vi "Add Buffers with Children.vi"(4 "channels":T1[](array[typedef]) {"string offset" format="%d bytes"}, 5 "inline":bool, 6 "Decimation":u64, 7 "Transfer Group Status":refnum<class "Status.lvclass">, 8 "error in (no error)":errorcluster, 9 "Buffers":refnum<class "Buffers.lvclass">, 10 "parent tag":string, 11 "Application Data In":T4) -> (0 "error out":errorcluster, 3 "Application Data out":T4)   [LabVIEW 2017, in "DSF Core.lvlib"]
uses:
  DSF Core.lvlib
  Main VI/Application Data.ctl
  <vilib>/NI/Memory Manager/Classes/Pointer/Pointer.lvclass
  Classes/Framework/Framework.lvclass
  Buffer Reader/Buffer Data.ctl
  Classes/Buffer/Buffer.lvclass
  C:/Program Files (x86)/National Instruments/LabVIEW 2017/vi.lib/NI/Memory Manager/Classes/Pointer/Pointer.lvclass
  Classes/Transfer Group Status/Status.lvclass
  Typedefs/DSF Engine Framework Configuration.ctl
  Typedefs/DSF Engine Plugin Configuration.ctl
  Typedefs/DSF Timing Info.ctl
  Typedefs/DSF Engine Plugin Thread Configuration.ctl
  Typedefs/DSF Settings Info.ctl
  Typedefs/DSF Engine Transfer Group Configuration.ctl
  Typedefs/DSF Direction.ctl
  Typedefs/DSF Engine Transfer Configuration.ctl
  Typedefs/DSF Byte Order.ctl
  Typedefs/DSF Engine Channel Configuration.ctl
  Typedefs/DSF Data Type.ctl
  Typedefs/DSF Timeout Behavior.ctl
  Classes/Buffers/Buffers.lvclass
  ID to Tree Items/Tree Item Type.ctl
  Classes/Buffers/Buffers.lvclass/Buffers.ctl
  <vilib>/NI/Memory Manager/Classes/Pointer/Pointer.lvclass/Pointer.ctl
  Classes/Buffer/Get Buffer Size.vi
  Sizeof.vi
  <vilib>/NI/Memory Manager/Classes/Pointer/Get Size.vi
  Classes/Buffer/Subset Buffer.vi
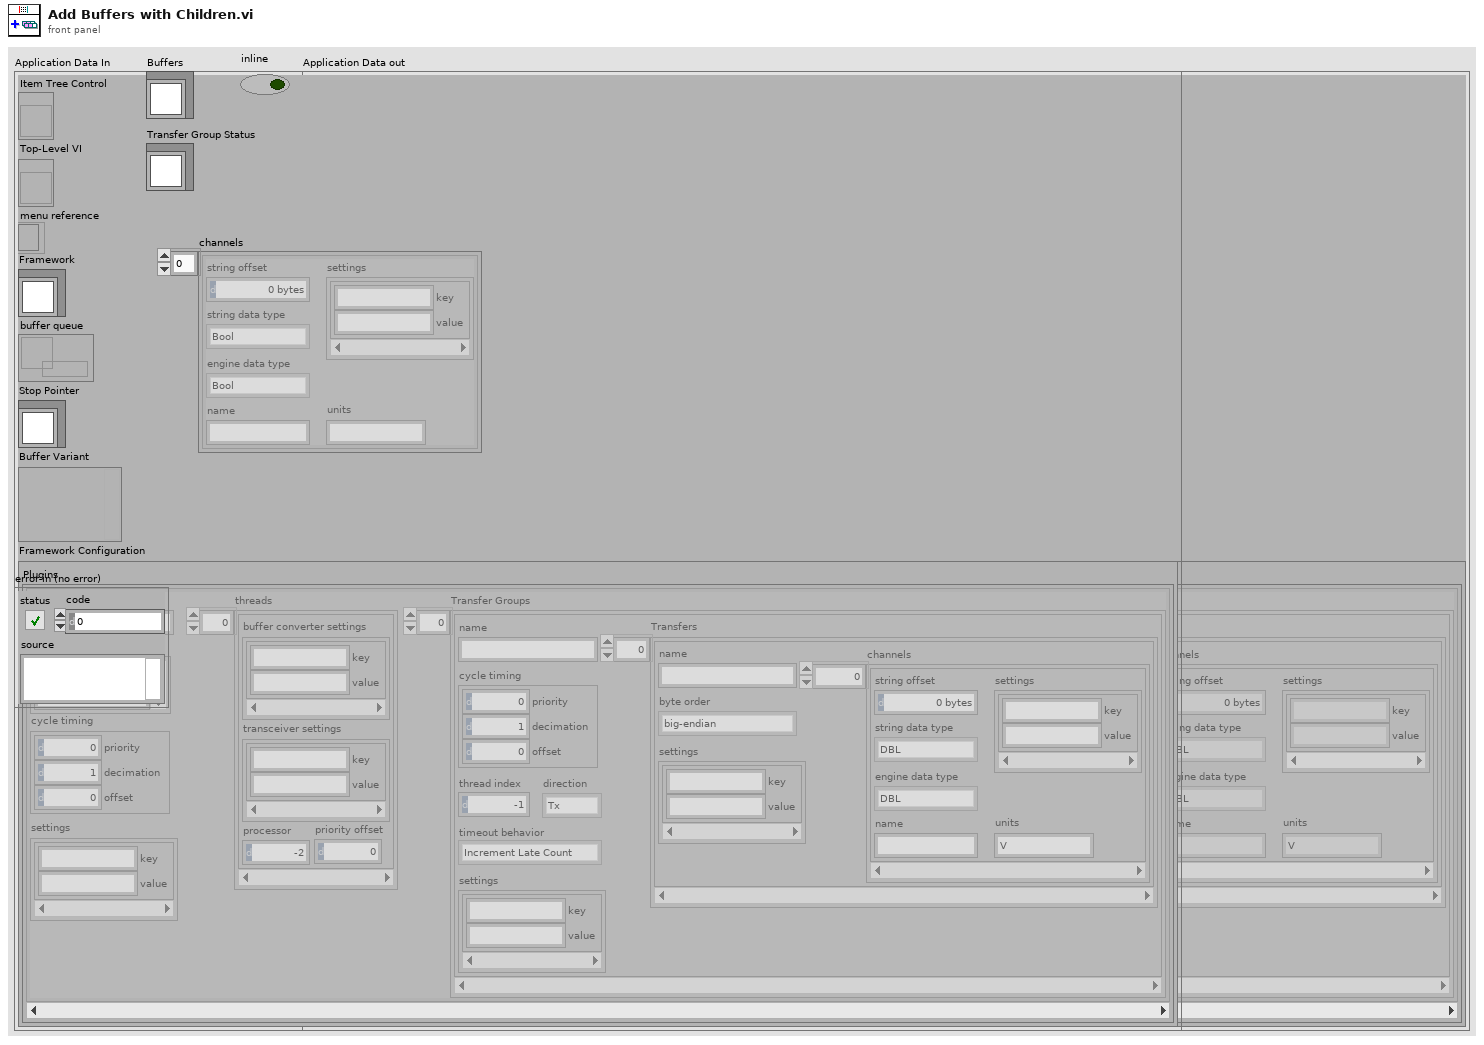
[diagram p1: front panel]
types:
  T1 = typedef "DSF Core.lvlib/DSF Engine Channel Configuration.ctl" = cluster{"string offset":u64, "string data type":T2, "engine data type":T2, "name":string, "settings":T3, "units":string}
  T2 = typedef "DSF Core.lvlib/DSF Data Type.ctl" = enum8{"Bool", "SGL", "DBL", "I8", "I16", "I32", "I64", "U8", "U16", "U32", "U64"}
  T3 = typedef "DSF Core.lvlib/DSF Settings Info.ctl" = cluster{"key":string, "value":string}[]
  T4 = typedef "DSF Core.lvlib/Application Data.ctl" = cluster{"Item Tree Control":refnum<vi>, "Top-Level VI":refnum<vi>, "menu reference":refnum<k9>, "Framework":refnum<class "Framework.lvclass">, "buffer queue":refnum<queue>, "Stop Pointer":refnum<class "Pointer.lvclass">, "Buffer Variant":variant, "Framework Configuration":T5}
  T5 = typedef "DSF Core.lvlib/DSF Engine Framework Configuration.ctl" = cluster{"Plugins":T6[]}
  T6 = typedef "DSF Core.lvlib/DSF Engine Plugin Configuration.ctl" = cluster{"name":string, "components":string[], "cycle timing":T7, "threads":T8[], "Transfer Groups":T9[], "settings":T3}
  T7 = typedef "DSF Core.lvlib/DSF Timing Info.ctl" = cluster{"priority":u64, "decimation":u64, "offset":u64}
  T8 = typedef "DSF Core.lvlib/DSF Engine Plugin Thread Configuration.ctl" = cluster{"buffer converter settings":T3, "transceiver settings":T3, "processor":i32, "priority offset":i16}
  T9 = typedef "DSF Core.lvlib/DSF Engine Transfer Group Configuration.ctl" = cluster{"name":string, "direction":T10, "cycle timing":T7, "thread index":i32, "settings":T3, "Transfers":T11[], "timeout behavior":T13}
  T10 = typedef "DSF Core.lvlib/DSF Direction.ctl" = enum8{"Tx", "Rx"}
  T11 = typedef "DSF Core.lvlib/DSF Engine Transfer Configuration.ctl" = cluster{"name":string, "byte order":T12, "settings":T3, "channels":T1[]}
  T12 = typedef "DSF Core.lvlib/DSF Byte Order.ctl" = enum8{"big-endian", "little-endian"}
  T13 = typedef "DSF Core.lvlib/DSF Timeout Behavior.ctl" = enum8{"Increment Late Count", "Throw Error"}
  T14 = typedef "DSF Core.lvlib/Buffer Data.ctl" = cluster{"Buffer":refnum<class "Buffer.lvclass">, "Status":refnum<class "Status.lvclass">, "decimation":u64, "avg bandwidth":dbl}
  T15 = typedef "DSF Core.lvlib/Tree Item Type.ctl" = enum16{"Framework", "Plugin Group", "Plugin", "Group", "Transfer", "Buffer", "Channel"}
  T16 = typedef "DSF Core.lvlib/Tree Item.ctl" = cluster{"Left Cell String":string, "Child Text":string[], "Child Tag":string, "Glyph Index":i32}
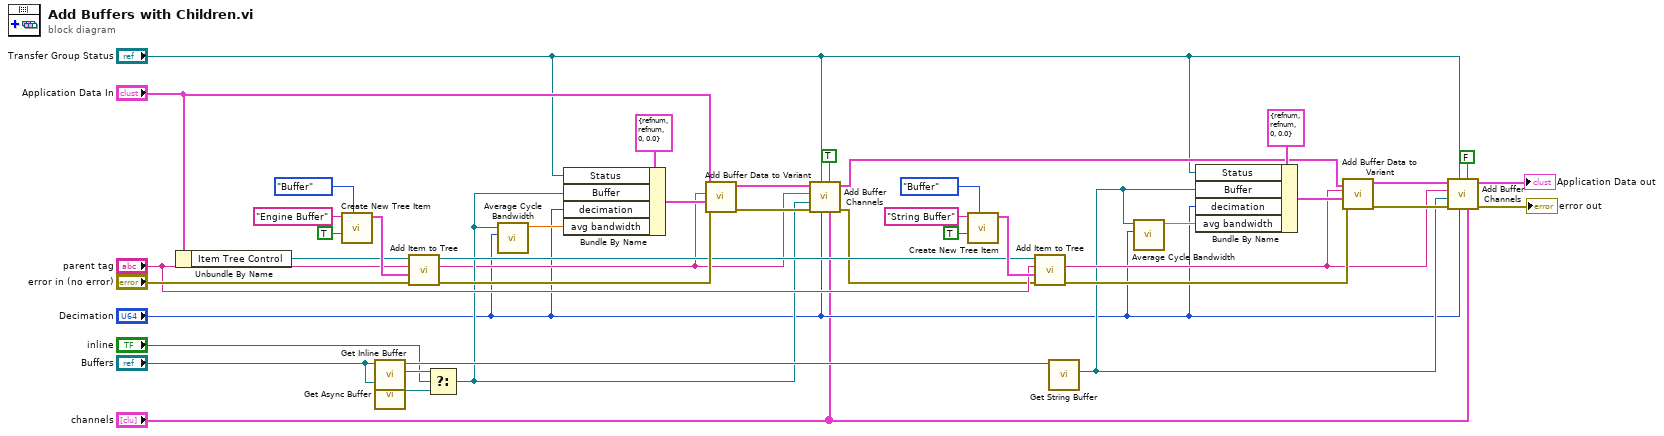
[diagram p0: block diagram]
diagram:
  n1 = Unbundle By Name("Application Data In") -> ("Item Tree Control"=w25:refnum<vi>)
  n2 = call "Create New Tree Item.vi"("Item Type"=Tree_Item_Type."Buffer", "found?"=TRUE, "Left Cell String"="Engine Buffer") -> ("Item"=w27:T16)  [unwired: 7 in, 1 out]
  n3 = call "Get Inline Buffer.vi"("Buffers in"="Buffers") -> ("Inline Buffer"=w19:refnum<class "Buffer.lvclass">, "Buffers out"=w34:refnum<class "Buffers.lvclass">)  [unwired: 9 in]
  n4 = call "Get Async Buffer.vi"("Buffers in"="Buffers") -> ("Async Buffer"=w20:refnum<class "Buffer.lvclass">)  [unwired: 9 in, 1 out]
  n5 = call "Add Item to Tree.vi"("error in (no error)"="error in (no error)", "Item"=w27, "parent tag"="parent tag", "TreeControl in"=w25) -> ("error out"=w40:errorcluster, "new item tag"=w12:string, "TreeControl out"=w35:refnum<vi>)  [unwired: 5 in]
  n6 = Select(t=w19, s="inline", f=w20) -> (s? t:f=w13:refnum<class "Buffer.lvclass">)
  n7 = call "Average Cycle Bandwidth.vi"("Decimation"="Decimation", "Buffer"=w13) -> ("avergage cycle bandwidth"=w23:dbl)  [unwired: 9 in]
  n8 = Bundle By Name(cluster=T14 {"Buffer"=refnum, "Status"=refnum, "decimation"=0, "avg bandwidth"=0.0} ("Buffer data"), "Status"="Transfer Group Status", "Buffer"=w13, "decimation"="Decimation", "avg bandwidth"=w23) -> (w39:T14)
  n9 = call "Add Buffer Data to Variant.vi"("error in (no error)"=w40, "Buffer data"=w39, "tag"=w12, "Application Data In in"="Application Data In") -> ("error out"=w15:errorcluster, "Application Data In out"=w17:T4)  [unwired: 6 in]
  n10 = call "Add Buffer Channels.vi"("channels"="channels", "engine (T) / string (F)"=TRUE, "Decimation"="Decimation", "Transfer Group Status"="Transfer Group Status", "error in (no error)"=w15, "Buffer"=w13, "parent tag"=w12, "Application Data In"=w17) -> ("error out"=w14:errorcluster, "Application Data out"=w16:T4)  [unwired: 2 in]
  n11 = call "Create New Tree Item.vi"("Item Type"=Tree_Item_Type."Buffer", "found?"=TRUE, "Left Cell String"="String Buffer") -> ("Item"=w36:T16)  [unwired: 7 in, 1 out]
  n12 = call "Add Item to Tree.vi"("error in (no error)"=w14, "Item"=w36, "parent tag"="parent tag", "TreeControl in"=w35) -> ("error out"=w43:errorcluster, "new item tag"=w6:string)  [unwired: 5 in, 1 out]
  n13 = call "Get String Buffer.vi"("Buffers in"=w34) -> ("String Buffer"=w5:refnum<class "Buffer.lvclass">)  [unwired: 9 in, 1 out]
  n14 = call "Average Cycle Bandwidth.vi"("Decimation"="Decimation", "Buffer"=w5) -> ("avergage cycle bandwidth"=w22:dbl)  [unwired: 9 in]
  n15 = Bundle By Name(cluster=T14 {"Buffer"=refnum, "Status"=refnum, "decimation"=0, "avg bandwidth"=0.0} ("Buffer data"), "Status"="Transfer Group Status", "Buffer"=w5, "decimation"="Decimation", "avg bandwidth"=w22) -> (w42:T14)
  n16 = call "Add Buffer Data to Variant.vi"("error in (no error)"=w43, "Buffer data"=w42, "tag"=w6, "Application Data In in"=w16) -> ("error out"=w8:errorcluster, "Application Data In out"=w10:T4)  [unwired: 6 in]
  n17 = call "Add Buffer Channels.vi"("channels"="channels", "engine (T) / string (F)"=FALSE, "Decimation"="Decimation", "Transfer Group Status"="Transfer Group Status", "error in (no error)"=w8, "Buffer"=w5, "parent tag"=w6, "Application Data In"=w10) -> ("error out"=→"error out":errorcluster, "Application Data out"=→"Application Data out":T4)  [unwired: 2 in]
